vi "AlliGator Enter Reference Lifetime Dialog.vi"(8 "Error In":errorcluster, 11 "Input Message":string="Enter phase lifetime to use as refrence:") -> (0 "Error Out":errorcluster, 1 "Cancelled?":bool, 3 "Reference Lifetime":dbl[unit])   [LabVIEW 2021, in "AlliGator Phasor Graph.lvlib"]
doc: "Reference Lifetime dialog."
uses:
  AlliGator Phasor Graph.lvlib
panel:
  in  "Reference Lifetime":dbl[unit] min=0.0 format="%.3g"
  in  "Cancel":bool
  in  "OK":bool
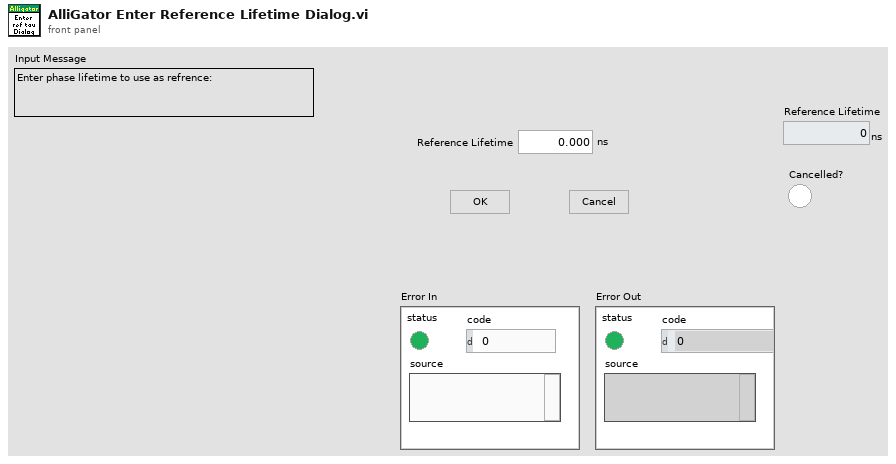
[diagram p1: front panel]
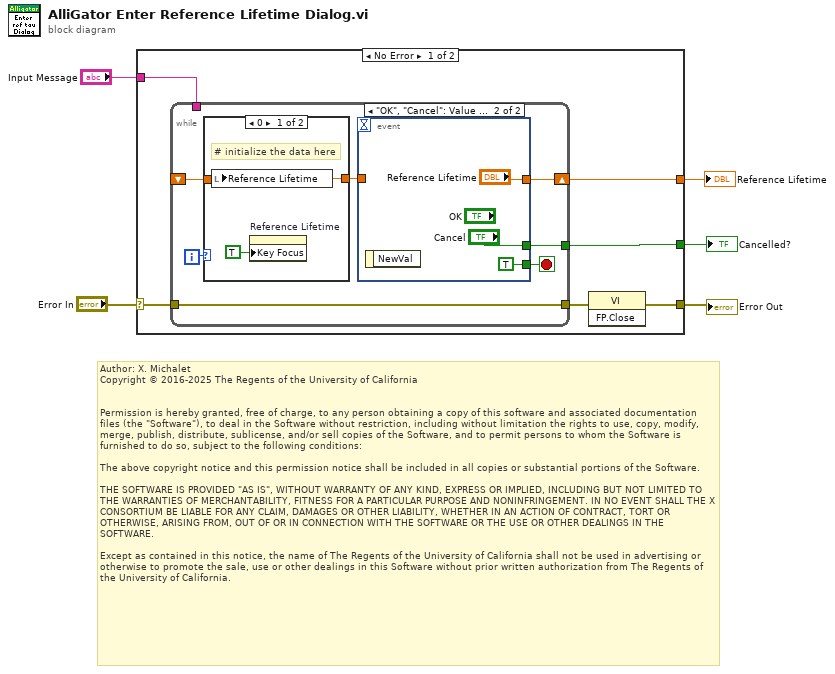
[diagram p0: block diagram]
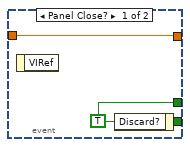
[diagram p3: hidden frame]
diagram:
  # "Author: X. Michalet\nCopyright © 2016-2025 The Regents of the University of California\n \n\nPermission is hereby granted, free of charge, to any person obtaining a copy of this software and associated documentation files (the \"Software\"), to deal in the Software without restriction, including without limitation the rights to use, copy, modify, merge, publish, distribute, sublicense, and/or sell copies of the Software, and to permit persons to whom the Software is furnished to do so, subject to the following conditions:\n\nThe above copyright notice and this permission notice shall be included in all copies or substantial portions of the Software.\n\nTHE SOFTWARE IS PROVIDED \"AS IS\", WITHOUT WARRANTY OF ANY KIND, EXPRESS OR IMPLIED, INCLUDING BUT NOT LIMITED TO THE WARRANTIES OF MERCHANTABILITY, FITNESS FOR A PARTICULAR PURPOSE AND NONINFRINGEMENT. IN NO EVENT SHALL THE X CONSORTIUM BE LIABLE FOR ANY CLAIM, DAMAGES OR OTHER LIABILITY, WHETHER IN AN ACTION OF CONTRACT, TORT OR OTHERWISE, ARISING FROM, OUT OF OR IN CONNECTION WITH THE SOFTWARE OR THE USE OR OTHER DEALINGS IN THE SOFTWARE.\n\nExcept as contained in this notice, the name of The Regents of the University of California shall not be used in advertising or otherwise to promote the sale, use or other dealings in this Software without prior written authorization from The Regents of the University of California."
  n1 = case shown="No Error" "Error In" {
    selector: "Error In" -> [w7 w27]
    tunnel: [w11 _] -> w5
    tunnel: [w10 _] -> w4
    tunnel: "Input Message" -> [w9 _]
    tunnel: [w8 w27] -> w1
    frame No Error {
      n2 = while {
        tunnel: [w17] -> w11
        shift-right: [w14] -> w10
        shift-left: _ -> [w15]
        tunnel: w9 -> [_]
        tunnel: w7 -> [w12]
        tunnel: [w12] -> w6
        i -> [w16]
        stop <- w18 stop-if-true
        n3 = case shown="0" w16 {
          tunnel: w15 -> [w20 w21]
          tunnel: [w20 w21] -> w13
          frame 0 {
            # "# initialize the data here"
            n4 = local write "Reference Lifetime"(w20) -> ()
            n5 = property on="Reference Lifetime" class="DigNum (strict)"("Key Focus"=TRUE) -> ()  [unwired: 2 in, 2 out]
          }
          frame 1, Default {
          }
        }
        n6 = event shown="[1] \"OK\", \"Cancel\": Value Change" {
          selector: _ -> [_ _]
          dyn-events: _ -> [_ _]
          timeout: _ -> [_ _]
          tunnel: [w23 TRUE ("Discard?")] -> w18
          tunnel: [w23 "Cancel"] -> w17
          tunnel: [w22 "Reference Lifetime"] -> w14
          tunnel: w13 -> [w22 _]
          event Panel Close? {
            w23 = TRUE ("Discard?")
            n7 = event-data() -> ()  [unwired: 1 in, 1 out]
            n8 = event-data("Discard?"=w23) -> ()  [unwired: 1 in, 1 out]
          }
          event "OK", "Cancel": Value Change {
            n9 = event-data() -> ()  [unwired: 1 in, 1 out]
          }
        }
      }
      n10 = invoke class="VI" method="FP.Close"(error in=w6) -> (error out=w8:errorcluster)  [unwired: 2 in, 2 out]
    }
    frame Error {
    }
  }
  "Reference Lifetime" <- w4
  "Cancelled?" <- w5
  "Error Out" <- w1
